vi "Count Actors.vi"(10 "Increment?":bool) -> ()   [LabVIEW 2020, in "Actor Framework.lvlib" / "Actor.lvclass"]
doc: "This VI compensates for a behavior of the LabVIEW runtime engine that is normally a feature but causes problems for a system as asynchronous as the Actor Framework. The usual rule for LabVIEW is that a VI can close its front panel and keep running as long as there is an open reference to a VI. However, in a runtime engine, if the very last front panel is closed, the application is immediately terminated. This was done as an aid to users who sometimes had runaway apps and no way to abort them other than the operating system kill switch. Actors, however, operate asynchronously, and sometimes the UI will shut down long before the other actors are finished. They may still be writing to configuration files or turning off hardware. There are also times when one UI will close and another open up, and we want the actors to proceed during the interim. Thus this VI exists. It opens its own front panel in the Hidden state, which is sufficient to keep LabVIEW from aborting all VIs and quitting. It counts how many actors have been launched and closes its panel after the last actor quits. Thus for applications using the Actor Framework, as long as even one actor is still running, the automatic abort behavior of the runtime engine will not occur."
uses:
  Actor.lvclass
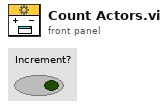
[diagram p1: front panel]
types:
  T1 = enum32{"Invalid", "Standard", "Closed", "Hidden", "Minimized", "Maximized"}
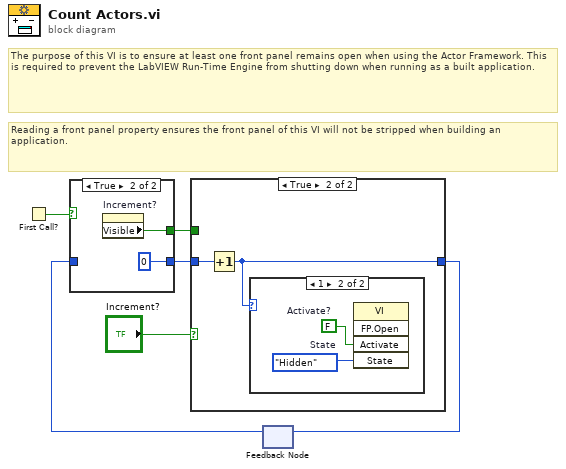
[diagram p0: block diagram]
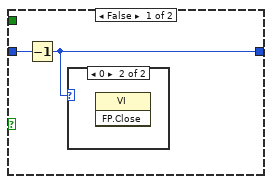
[diagram p2: hidden frame]
diagram:
  # "Reading a front panel property ensures the front panel of this VI will not be stripped when building an application."
  # "The purpose of this VI is to ensure at least one front panel remains open when using the Actor Framework. This is required to prevent the LabVIEW Run-Time Engine from shutting down when running as a built application."
  n1 = First Call?() -> (First Call?: T/F=w5:bool)
  n2 = feedback #1() -> (w2:u32)  [unwired: 1 in]
  n3 = case shown="True" w5 {
    tunnel: w2 -> [w7 _]
    tunnel: [w7 u32 0] -> w4
    tunnel: [_ w8] -> w1
    frame False {
    }
    frame True {
      n4 = property on="Increment?" class="Bool (strict)"() -> ("Visible"=w8:bool)  [unwired: 2 in, 2 out]
    }
  }
  n5 = case shown="True" "Increment?" {
    tunnel: w4 -> [w11 w13]
    tunnel: [w10 w12] -> w3
    tunnel: w1 -> [_ _]
    frame False {
      n6 = Decrement(x=w11) -> (x-1=w10:u32)
      n7 = case shown="0" w10 {
        frame Default {
        }
        frame 0 {
          n8 = invoke class="VI" method="FP.Close"() -> ()  [unwired: 3 in, 3 out]
        }
      }
    }
    frame True {
      n9 = Increment(x=w13) -> (x+1=w12:u32)
      n10 = case shown="1" w12 {
        frame Default {
        }
        frame 1 {
          w14 = FALSE  # Activate?
          w15 = T1."Hidden"  # State
          n11 = invoke class="VI" method="FP.Open"("Activate"=w14, "State"=w15) -> ()  [unwired: 3 in, 5 out]
        }
      }
    }
  }
  n12 = feedback-in #1(w3) -> ()
